vi "While Loop Stop with Nested Conditionals Example.vi"() -> ()   [LabVIEW 2020, in "Test Executive.lvlib" / "Nested Conditional in While Loop Example.lvlib"]
uses:
  <vilib>/gpm_packages/@cs/test-executive/Source/Sandbox/Nested Conditional in While Loop Example/Nested Conditional in While Loop Example.lvlib
  <vilib>/gpm_packages/@cs/test-executive/Source/Test Executive/TestExecutive/Test Executive.lvclass
  C:/Program Files/National Instruments/LabVIEW 2020/vi.lib/gpm_packages/@cs/test-executive/Source/Test Executive/ITestExecutive/ITest Executive.lvclass
  <vilib>/gpm_packages/@cs/test-executive/Source/Sandbox/Nested Conditional in While Loop Example/Device End Finder/Device End Finder.lvclass
  <vilib>/gpm_packages/@cs/test-executive/Source/Sandbox/Nested Conditional in While Loop Example/iTest Step/iTest Step.lvclass
  <vilib>/gpm_packages/@cs/test-executive/Source/Sandbox/Nested Conditional in While Loop Example/Device Post Dip Length/Device Post Dip Length.lvclass
  <vilib>/gpm_packages/@cs/test-executive/Source/Sandbox/Nested Conditional in While Loop Example/Iterate/Iterate.lvclass
  <vilib>/gpm_packages/@cs/run-time-assertions/Source/Assert Less/Assert Less.lvclass
  C:/Program Files/National Instruments/LabVIEW 2020/vi.lib/gpm_packages/@cs/run-time-assertions/Source/Assert/Assert.lvclass
  <vilib>/gpm_packages/@cs/run-time-assertions/Source/Assert Greater or Equal/Assert Greater or Equal.lvclass
  52cc7c55-fdef-40cb-9b01-06c8b27f6ce0.vi
  a0d94dfd-d8d0-4b1a-8204-38a80b6efbaa.vi
  22f6ace6-23ce-4251-a6e4-277f1b0ddc71.vi
  5f10894d-39a4-4711-8d45-a7dfc19e406e.vi
  be74f702-6a90-4609-b438-3fe557b35d77.vi
  a10d8200-898b-41a6-a462-7d6528bd6408.vi
  f7a3b14d-821f-4fd9-982f-4d6d978a7b0b.vi
  0ece8d78-e94c-4796-b66e-215c9e74c0e8.vi
  0df7ce8f-9091-4b2d-8a2a-2bb6b5b20627.vi
  b94ec968-1831-4c86-b0ad-5031bb25da7e.vi
  78029b1d-24e3-44ce-bc53-a6c931d15c9f.vi
  <vilib>/Utility/error.llb/Error Cluster From Error Code.vi
  <vilib>/gpm_packages/@cs/test-executive/Source/Test Executive/ITestExecutive/ITest Executive.lvclass
  <vilib>/gpm_packages/@cs/test-executive/Source/Test Executive/TestExecutive Ref/TestExecutive Ref.lvclass
  <vilib>/gpm_packages/@cs/test-executive/Source/Test Executive/Executioner/Executioner.lvclass
panel:
  in  "Stop":bool
  in  "Tree":string(tree)
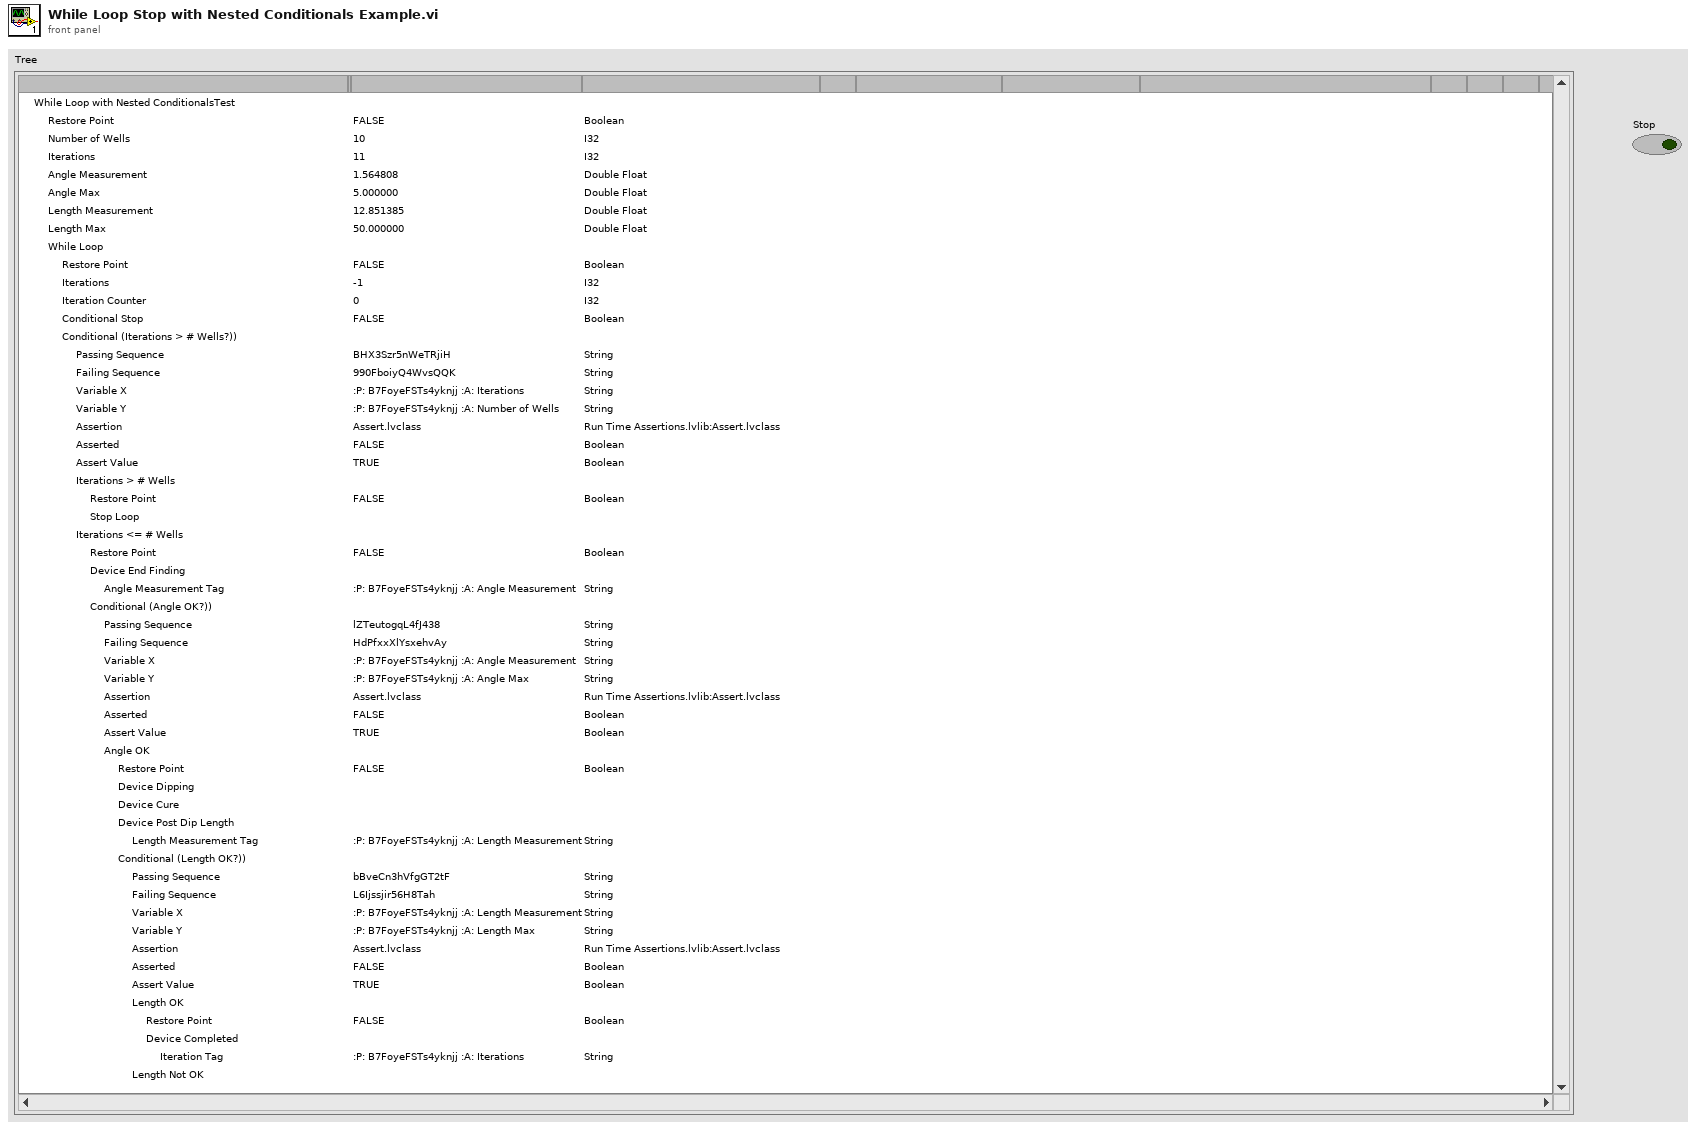
[diagram p1: front panel]
types:
  T1 = cluster{"Left Cell String":string, "Child Text":string[], "Child Tag":string, "Item Indent":i32, "Child Only?":bool, "Glyph Index":i32}[]
diagram:
  n1 = flat-sequence {
    tunnel: [w184] -> w181
    tunnel: [w183] -> w180
    tunnel: [w182] -> w168
    frame #0 {
      # "Create Test Executive"
      n2 = call <vilib>:"Create New Test Executive.vi"("Name"="While Loop with Nested ConditionalsTest", "Test Executive"=refnum<class "Test Executive.lvclass"> refnum ("Test Executive.lvlib:Test Executive.lvclass")) -> ("error out"=w183:errorcluster, "Test Executive Ref"=w184:refnum<data-value>, "Test Executive ID out"=w182:string)  [unwired: 7 in]
    }
  }
  n3 = flat-sequence {
    tunnel: w181 -> [w198]
    tunnel: w180 -> [w197]
    tunnel: [w191] -> w165
    tunnel: [w190] -> w166
    tunnel: [w189] -> w170
    tunnel: [w188] -> w169
    tunnel: w168 -> [w187]
    tunnel: [w187] -> w167
    frame #0 {
      # "Create attributes for stopping top level loop"
      n4 = call "Add Attribute.vim"("ID"=w187, "error in (no error)"=w197, "Attribute"=10, "Attribute Name"="Number of Wells", "Test Executive Ref"=w198) -> ("error out"=w192:errorcluster, "Attribute ID out"=w191:string, "Test Executive Ref out"=w193:refnum<data-value>)  [unwired: 3 in, 1 out]
      n5 = call "Add Attribute.vim"("ID"=w187, "error in (no error)"=w192, "Attribute"=0, "Attribute Name"="Iterations", "Test Executive Ref"=w193) -> ("error out"=w188:errorcluster, "Attribute ID out"=w190:string, "Test Executive Ref out"=w189:refnum<data-value>)  [unwired: 3 in, 1 out]
    }
  }
  n6 = flat-sequence {
    tunnel: w170 -> [w212]
    tunnel: [w205] -> w159
    tunnel: w169 -> [w211]
    tunnel: [w203] -> w157
    tunnel: w167 -> [w202]
    tunnel: [w202] -> w164
    tunnel: [w210] -> w162
    tunnel: w166 -> [w210]
    tunnel: [w209] -> w163
    tunnel: w165 -> [w209]
    tunnel: [w201] -> w161
    tunnel: [w200] -> w160
    frame #0 {
      # "Create attributes for Angle OK evaluation\nNote that we are just creating a made up Angle Max that we can use for comparison purposes in the conditional"
      n7 = call "Add Attribute.vim"("ID"=w202, "error in (no error)"=w211, "Attribute"=0.0, "Attribute Name"="Angle Measurement", "Test Executive Ref"=w212) -> ("error out"=w204:errorcluster, "Attribute ID out"=w201:string, "Test Executive Ref out"=w206:refnum<data-value>)  [unwired: 3 in, 1 out]
      n8 = call "Add Attribute.vim"("ID"=w202, "error in (no error)"=w204, "Attribute"=5.0, "Attribute Name"="Angle Max", "Test Executive Ref"=w206) -> ("error out"=w203:errorcluster, "Attribute ID out"=w200:string, "Test Executive Ref out"=w205:refnum<data-value>)  [unwired: 3 in, 1 out]
    }
  }
  n9 = flat-sequence {
    tunnel: [w226] -> w158
    tunnel: [w224] -> w156
    tunnel: [w221] -> w155
    tunnel: [w219] -> w154
    tunnel: [w220] -> w153
    tunnel: [w223] -> w150
    tunnel: [w222] -> w149
    tunnel: w164 -> [w221]
    tunnel: w163 -> [w220]
    tunnel: w162 -> [w219]
    tunnel: [w218] -> w152
    tunnel: w161 -> [w218]
    tunnel: [w217] -> w151
    tunnel: w160 -> [w217]
    tunnel: w159 -> [w216]
    tunnel: w157 -> [w215]
    frame #0 {
      # "Create attributes for Length OK evaluation\nNote that we are just creating a made up Length Max that we can use for comparison purposes in the conditional"
      n10 = call "Add Attribute.vim"("ID"=w221, "error in (no error)"=w215, "Attribute"=0.0, "Attribute Name"="Length Measurement", "Test Executive Ref"=w216) -> ("error out"=w225:errorcluster, "Attribute ID out"=w223:string, "Test Executive Ref out"=w227:refnum<data-value>)  [unwired: 3 in, 1 out]
      n11 = call "Add Attribute.vim"("ID"=w221, "error in (no error)"=w225, "Attribute"=50.0, "Attribute Name"="Length Max", "Test Executive Ref"=w227) -> ("error out"=w224:errorcluster, "Attribute ID out"=w222:string, "Test Executive Ref out"=w226:refnum<data-value>)  [unwired: 3 in, 1 out]
    }
  }
  n12 = flat-sequence {
    tunnel: [w243] -> w179
    tunnel: [w242] -> w178
    tunnel: [w241] -> w145
    tunnel: w155 -> [w232]
    tunnel: w158 -> [w240]
    tunnel: w156 -> [w239]
    tunnel: [w232] -> w148
    tunnel: [w238] -> w147
    tunnel: w154 -> [w238]
    tunnel: [w237] -> w146
    tunnel: w153 -> [w237]
    tunnel: w152 -> [w236]
    tunnel: w151 -> [w235]
    tunnel: w150 -> [w234]
    tunnel: w149 -> [w233]
    tunnel: [w236] -> w141
    tunnel: [w235] -> w142
    tunnel: [w234] -> w143
    tunnel: [w233] -> w144
    frame #0 {
      # "Create While Loop"
      n13 = call <vilib>:"Insert While Loop.vi"("Parent ID"=w232, "error in (no error)"=w239, "Name"="While Loop", "Test Executive Ref"=w240) -> ("error out"=w242:errorcluster, "Test Executive Ref out"=w243:refnum<data-value>, "Unique ID out"=w241:string)  [unwired: 4 in, 1 out]
    }
  }
  n14 = flat-sequence {
    tunnel: w179 -> [w261]
    tunnel: w178 -> [w260]
    tunnel: w145 -> [w249]
    tunnel: [w257] -> w177
    tunnel: [w255] -> w176
    tunnel: [w254] -> w138
    tunnel: [w252] -> w140
    tunnel: w148 -> [w252]
    tunnel: [w251] -> w136
    tunnel: w147 -> [w251]
    tunnel: w146 -> [w250]
    tunnel: [w250] -> w137
    tunnel: [w249] -> w139
    tunnel: [w248] -> w132
    tunnel: w144 -> [w248]
    tunnel: [w247] -> w133
    tunnel: w143 -> [w247]
    tunnel: [w246] -> w134
    tunnel: w142 -> [w246]
    tunnel: [w245] -> w135
    tunnel: w141 -> [w245]
    frame #0 {
      # "Create True Conditional Branch and nest a Stop Loop\nThis branch executes when Iterations > # wells"
      n15 = call <vilib>:"Insert Conditional Branch.vi"("Parent ID"=w249, "error in (no error)"=w260, "Name"="Iterations > # Wells", "Test Executive Ref"=w261) -> ("error out"=w256:errorcluster, "Test Executive Ref out"=w258:refnum<data-value>, "Unique ID out"=w254:string)  [unwired: 4 in, 1 out]
      n16 = call <vilib>:"Insert Stop Loop.vi"("Parent ID"=w254, "error in (no error)"=w256, "Name"="Stop Loop", "Test Executive Ref"=w258) -> ("error out"=w255:errorcluster, "Test Executive Ref out"=w257:refnum<data-value>)  [unwired: 4 in, 2 out]
    }
  }
  n17 = flat-sequence {
    tunnel: w177 -> [w275]
    tunnel: w176 -> [w274]
    tunnel: [w263] -> w70
    tunnel: [w262] -> w69
    tunnel: [w273] -> w71
    tunnel: w139 -> [w271]
    tunnel: [w272] -> w73
    tunnel: w140 -> [w272]
    tunnel: [w271] -> w72
    tunnel: [w270] -> w62
    tunnel: w138 -> [w270]
    tunnel: w137 -> [w269]
    tunnel: [w269] -> w63
    tunnel: [w268] -> w64
    tunnel: w136 -> [w268]
    tunnel: [w267] -> w65
    tunnel: w135 -> [w267]
    tunnel: [w266] -> w66
    tunnel: w134 -> [w266]
    tunnel: [w265] -> w67
    tunnel: w133 -> [w265]
    tunnel: [w264] -> w68
    tunnel: w132 -> [w264]
    frame #0 {
      # "Create False Conditional Branch\nThis branch exectues when Iterations <= # Wells"
      n18 = call <vilib>:"Insert Conditional Branch.vi"("Parent ID"=w271, "error in (no error)"=w274, "Name"="Iterations <= # Wells", "Test Executive Ref"=w275) -> ("error out"=w262:errorcluster, "Test Executive Ref out"=w263:refnum<data-value>, "Unique ID out"=w273:string)  [unwired: 4 in, 1 out]
    }
  }
  n19 = flat-sequence {
    tunnel: w70 -> [w294]
    tunnel: [w293] -> w129
    tunnel: w69 -> [w292]
    tunnel: [w291] -> w128
    tunnel: w71 -> [w287]
    tunnel: [w289] -> w123
    tunnel: w73 -> [w289]
    tunnel: [w288] -> w122
    tunnel: w72 -> [w288]
    tunnel: [w287] -> w130
    tunnel: [w286] -> w120
    tunnel: w64 -> [w286]
    tunnel: [w285] -> w119
    tunnel: w63 -> [w285]
    tunnel: [w284] -> w118
    tunnel: w62 -> [w284]
    tunnel: w65 -> [w283]
    tunnel: w66 -> [w282]
    tunnel: w67 -> [w281]
    tunnel: w68 -> [w280]
    tunnel: [w283] -> w124
    tunnel: [w282] -> w125
    tunnel: [w281] -> w126
    tunnel: [w280] -> w127
    tunnel: [w277] -> w131
    frame #0 {
      # "Device End Finding\nThis should generate an Angle measurement"
      n20 = call <vilib>:"Create Test from Object.vi"("Test"=refnum<class "Device End Finder.lvclass"> refnum ("Nested Conditional in While Loop Example.lvlib:Device End Finder.lvclass")) -> ("Test"=w279:refnum<class "Executioner.lvclass">)  [unwired: 10 in]
      n21 = call <vilib>:"Insert Test.vi"("Parent ID"=w287, "error in (no error)"=w292, "Test"=w279, "Name"="Device End Finding", "Test Executive Ref"=w294) -> ("error out"=w291:errorcluster, "Test Executive Ref out"=w293:refnum<data-value>, "Unique ID out"=w277:string)  [unwired: 3 in, 1 out]
    }
  }
  n22 = flat-sequence {
    tunnel: w129 -> [w310]
    tunnel: w128 -> [w309]
    tunnel: w131 -> [w308]
    tunnel: [w306] -> _
    tunnel: [w305] -> _
    tunnel: w120 -> [w299]
    tunnel: [w304] -> _
    tunnel: w123 -> [w304]
    tunnel: [w296] -> _
    tunnel: [w296] -> _
    tunnel: [w303] -> w121
    tunnel: w130 -> [w303]
    tunnel: [w302] -> w114
    tunnel: w127 -> [w302]
    tunnel: [w301] -> w115
    tunnel: w126 -> [w301]
    tunnel: [w300] -> w116
    tunnel: w125 -> [w300]
    tunnel: w124 -> [w295]
    tunnel: [w299] -> _
    tunnel: [w298] -> _
    tunnel: w118 -> [w298]
    tunnel: [w297] -> _
    tunnel: w119 -> [w297]
    tunnel: [w295] -> w117
    tunnel: w122 -> [w296]
    frame #0 {
      # "Insert an attribute that holds the\ntag for the variable we want to\nstore angle measurement in"
      n23 = call "Add Attribute.vim"("ID"=w308, "error in (no error)"=w309, "Attribute"=w295, "Attribute Name"="Angle Measurement Tag", "Test Executive Ref"=w310) -> ("error out"=w305:errorcluster, "Test Executive Ref out"=w306:refnum<data-value>)  [unwired: 3 in, 2 out]
    }
  }
  n24 = flat-sequence {
    tunnel: [w318] -> w109
    tunnel: [w315] -> w108
    tunnel: w121 -> [w331]
    tunnel: w129 -> [w335]
    tunnel: w128 -> [w334]
    tunnel: [w333] -> w113
    tunnel: w123 -> [w333]
    tunnel: [w332] -> w112
    tunnel: w122 -> [w332]
    tunnel: [w331] -> w111
    tunnel: [w330] -> w105
    tunnel: w120 -> [w330]
    tunnel: w119 -> [w311]
    tunnel: [w329] -> w107
    tunnel: w118 -> [w329]
    tunnel: [w328] -> w104
    tunnel: w117 -> [w328]
    tunnel: [w327] -> w103
    tunnel: w116 -> [w327]
    tunnel: [w326] -> w102
    tunnel: w115 -> [w326]
    tunnel: [w325] -> w101
    tunnel: w114 -> [w325]
    tunnel: [w314] -> w110
    tunnel: [w311] -> w106
    frame #0 {
      # "This branch executes when Angle measurement after Device End Finding returns as OK\nInsert some dummy test steps that match the flow chart"
      n25 = call <vilib>:"Insert Conditional Branch.vi"("Parent ID"=w331, "error in (no error)"=w334, "Name"="Angle OK", "Test Executive Ref"=w335) -> ("error out"=w317:errorcluster, "Test Executive Ref out"=w320:refnum<data-value>, "Unique ID out"=w314:string)  [unwired: 4 in, 1 out]
      n26 = call <vilib>:"Create Test from Object.vi"("Test"=refnum<class "iTest Step.lvclass"> refnum ("Nested Conditional in While Loop Example.lvlib:iTest Step.lvclass")) -> ("Test"=w324:refnum<class "Executioner.lvclass">)  [unwired: 10 in]
      n27 = call <vilib>:"Insert Test.vi"("Parent ID"=w314, "error in (no error)"=w317, "Test"=w324, "Name"="Device Dipping", "Test Executive Ref"=w320) -> ("error out"=w316:errorcluster, "Test Executive Ref out"=w319:refnum<data-value>)  [unwired: 3 in, 2 out]
      n28 = call <vilib>:"Create Test from Object.vi"("Test"=refnum<class "iTest Step.lvclass"> refnum ("Nested Conditional in While Loop Example.lvlib:iTest Step.lvclass")) -> ("Test"=w321:refnum<class "Executioner.lvclass">)  [unwired: 10 in]
      n29 = call <vilib>:"Insert Test.vi"("Parent ID"=w314, "error in (no error)"=w316, "Test"=w321, "Name"="Device Cure", "Test Executive Ref"=w319) -> ("error out"=w315:errorcluster, "Test Executive Ref out"=w318:refnum<data-value>)  [unwired: 3 in, 2 out]
    }
  }
  n30 = flat-sequence {
    tunnel: w109 -> [w355]
    tunnel: [w354] -> w95
    tunnel: w108 -> [w353]
    tunnel: [w352] -> w94
    tunnel: w111 -> [w340]
    tunnel: [w350] -> w100
    tunnel: w113 -> [w350]
    tunnel: [w349] -> w99
    tunnel: w112 -> [w349]
    tunnel: [w340] -> w98
    tunnel: [w348] -> w89
    tunnel: w105 -> [w348]
    tunnel: [w347] -> w88
    tunnel: w106 -> [w347]
    tunnel: [w346] -> w87
    tunnel: w107 -> [w346]
    tunnel: w104 -> [w345]
    tunnel: w103 -> [w344]
    tunnel: w102 -> [w343]
    tunnel: w101 -> [w342]
    tunnel: [w345] -> w90
    tunnel: [w344] -> w91
    tunnel: [w343] -> w92
    tunnel: [w342] -> w93
    tunnel: w110 -> [w339]
    tunnel: [w339] -> w97
    tunnel: [w338] -> w96
    frame #0 {
      # "Device End Finding\nThis should generate an Angle measurement"
      n31 = call <vilib>:"Create Test from Object.vi"("Test"=refnum<class "Device Post Dip Length.lvclass"> refnum ("Nested Conditional in While Loop Example.lvlib:Device Post Dip Length.lvclass")) -> ("Test"=w341:refnum<class "Executioner.lvclass">)  [unwired: 10 in]
      n32 = call <vilib>:"Insert Test.vi"("Parent ID"=w339, "error in (no error)"=w353, "Test"=w341, "Name"="Device Post Dip Length", "Test Executive Ref"=w355) -> ("error out"=w352:errorcluster, "Test Executive Ref out"=w354:refnum<data-value>, "Unique ID out"=w338:string)  [unwired: 3 in, 1 out]
    }
  }
  n33 = flat-sequence {
    tunnel: [w372] -> w86
    tunnel: w100 -> [w372]
    tunnel: [w371] -> w85
    tunnel: w99 -> [w371]
    tunnel: [w370] -> w84
    tunnel: w98 -> [w370]
    tunnel: [w358] -> w83
    tunnel: w97 -> [w358]
    tunnel: [w362] -> w82
    tunnel: w95 -> [w363]
    tunnel: [w360] -> w81
    tunnel: w94 -> [w361]
    tunnel: [w369] -> w74
    tunnel: w93 -> [w369]
    tunnel: [w357] -> w75
    tunnel: w92 -> [w357]
    tunnel: w91 -> [w368]
    tunnel: [w368] -> w76
    tunnel: w90 -> [w367]
    tunnel: [w367] -> w77
    tunnel: [w366] -> w80
    tunnel: w87 -> [w366]
    tunnel: [w365] -> w79
    tunnel: w88 -> [w365]
    tunnel: [w364] -> w78
    tunnel: w89 -> [w364]
    tunnel: w96 -> [w356]
    frame #0 {
      # "Insert an attribute that holds the\ntag for the variable we want to\nstore length measurement in"
      n34 = call "Add Attribute.vim"("ID"=w356, "error in (no error)"=w361, "Attribute"=w357, "Attribute Name"="Length Measurement Tag", "Test Executive Ref"=w363) -> ("error out"=w360:errorcluster, "Test Executive Ref out"=w362:refnum<data-value>)  [unwired: 3 in, 2 out]
    }
  }
  n35 = flat-sequence {
    tunnel: [w398] -> w51
    tunnel: w86 -> [w398]
    tunnel: [w397] -> w50
    tunnel: w85 -> [w397]
    tunnel: [w387] -> w49
    tunnel: w84 -> [w387]
    tunnel: w83 -> [w376]
    tunnel: w82 -> [w393]
    tunnel: w81 -> [w392]
    tunnel: [w378] -> w54
    tunnel: w78 -> [w378]
    tunnel: [w396] -> w53
    tunnel: w79 -> [w396]
    tunnel: [w395] -> w52
    tunnel: w80 -> [w395]
    tunnel: w77 -> [w384]
    tunnel: w76 -> [w385]
    tunnel: w75 -> [w377]
    tunnel: w74 -> [w386]
    tunnel: [w386] -> w58
    tunnel: [w377] -> w57
    tunnel: [w385] -> w56
    tunnel: [w384] -> w55
    tunnel: [w376] -> w61
    tunnel: [w375] -> w60
    tunnel: [w374] -> w59
    tunnel: [w373] -> w43
    frame #0 {
      # "This is the branch that will execute when the length measurement is OK.\nIt will call the Device Completed test step, which runs a dummy step that will increment the counter"
      n36 = call <vilib>:"Insert Conditional Branch.vi"("Parent ID"=w376, "error in (no error)"=w392, "Name"="Length OK", "Test Executive Ref"=w393) -> ("error out"=w388:errorcluster, "Test Executive Ref out"=w389:refnum<data-value>, "Unique ID out"=w373:string)  [unwired: 4 in, 1 out]
      n37 = call <vilib>:"Create Test from Object.vi"("Test"=refnum<class "Iterate.lvclass"> refnum ("Nested Conditional in While Loop Example.lvlib:Iterate.lvclass")) -> ("Test"=w390:refnum<class "Executioner.lvclass">)  [unwired: 10 in]
      n38 = call <vilib>:"Insert Test.vi"("Parent ID"=w373, "error in (no error)"=w388, "Test"=w390, "Name"="Device Completed", "Test Executive Ref"=w389) -> ("error out"=w380:errorcluster, "Test Executive Ref out"=w381:refnum<data-value>, "Unique ID out"=w379:string)  [unwired: 3 in, 1 out]
      n39 = call "Add Attribute.vim"("ID"=w379, "error in (no error)"=w380, "Attribute"=w378, "Attribute Name"="Iteration Tag", "Test Executive Ref"=w381) -> ("error out"=w374:errorcluster, "Test Executive Ref out"=w375:refnum<data-value>)  [unwired: 3 in, 2 out]
    }
  }
  n40 = flat-sequence {
    tunnel: [w425] -> w40
    tunnel: w51 -> [w425]
    tunnel: [w424] -> w39
    tunnel: w50 -> [w424]
    tunnel: [w414] -> w38
    tunnel: w49 -> [w414]
    tunnel: w61 -> [w403]
    tunnel: w60 -> [w420]
    tunnel: w59 -> [w419]
    tunnel: [w405] -> w35
    tunnel: w54 -> [w405]
    tunnel: [w423] -> w34
    tunnel: w53 -> [w423]
    tunnel: [w422] -> w33
    tunnel: w52 -> [w422]
    tunnel: w55 -> [w411]
    tunnel: w56 -> [w412]
    tunnel: w57 -> [w404]
    tunnel: w58 -> [w413]
    tunnel: [w413] -> w47
    tunnel: [w404] -> w48
    tunnel: [w412] -> w37
    tunnel: [w411] -> w36
    tunnel: [w403] -> w44
    tunnel: [w402] -> w46
    tunnel: [w401] -> w45
    tunnel: w43 -> [w400]
    tunnel: [w400] -> w42
    tunnel: [w399] -> w41
    frame #0 {
      # "This is the branch that will execute when the length measurement is not OK.\nIt will call the Device Rejection test step, which runs a dummy step that will increment the counter"
      n41 = call <vilib>:"Insert Conditional Branch.vi"("Parent ID"=w403, "error in (no error)"=w419, "Name"="Length Not OK", "Test Executive Ref"=w420) -> ("error out"=w415:errorcluster, "Test Executive Ref out"=w416:refnum<data-value>, "Unique ID out"=w399:string)  [unwired: 4 in, 1 out]
      n42 = call <vilib>:"Create Test from Object.vi"("Test"=refnum<class "Iterate.lvclass"> refnum ("Nested Conditional in While Loop Example.lvlib:Iterate.lvclass")) -> ("Test"=w417:refnum<class "Executioner.lvclass">)  [unwired: 10 in]
      n43 = call <vilib>:"Insert Test.vi"("Parent ID"=w399, "error in (no error)"=w415, "Test"=w417, "Name"="Device Rejection", "Test Executive Ref"=w416) -> ("error out"=w407:errorcluster, "Test Executive Ref out"=w408:refnum<data-value>, "Unique ID out"=w406:string)  [unwired: 3 in, 1 out]
      n44 = call "Add Attribute.vim"("ID"=w406, "error in (no error)"=w407, "Attribute"=w405, "Attribute Name"="Iteration Tag", "Test Executive Ref"=w408) -> ("error out"=w401:errorcluster, "Test Executive Ref out"=w402:refnum<data-value>)  [unwired: 3 in, 2 out]
    }
  }
  n45 = flat-sequence {
    tunnel: w48 -> [w443]
    tunnel: w47 -> [w442]
    tunnel: w46 -> [w440]
    tunnel: w45 -> [w439]
    tunnel: w44 -> [w426]
    tunnel: w42 -> [w438]
    tunnel: w41 -> [w437]
    tunnel: [w436] -> w32
    tunnel: w40 -> [w436]
    tunnel: [w435] -> w31
    tunnel: w39 -> [w435]
    tunnel: [w434] -> w30
    tunnel: w38 -> [w434]
    tunnel: w37 -> [w433]
    tunnel: w36 -> [w432]
    tunnel: [w433] -> w27
    tunnel: [w432] -> w26
    tunnel: [w431] -> w23
    tunnel: w35 -> [w431]
    tunnel: w34 -> [w430]
    tunnel: [w430] -> w24
    tunnel: w33 -> [w429]
    tunnel: [w429] -> w25
    tunnel: [w428] -> w29
    tunnel: [w427] -> w28
    tunnel: [w426] -> w22
    frame #0 {
      # "Setup the conditional inside the Length OK Branch"
      n46 = call <vilib>:"Insert Conditional.vi"("Test Executive Ref"=w440, "Name"="Conditional (Length OK?))", "Assertion"=refnum<class "Assert Less.lvclass"> refnum ("Run Time Assertions.lvlib:Assert Less.lvclass"), "error in (no error)"=w439, "Parent ID"=w426, "Variable X"=w443, "Variable Y"=w442, "Passing Executive"=w438, "Failing Executive"=w437) -> ("Test Executive Ref out"=w428:refnum<data-value>, "error out"=w427:errorcluster)  [unwired: 7 in, 2 out]
    }
  }
  n47 = flat-sequence {
    tunnel: [w449] -> w20
    tunnel: [w447] -> w18
    tunnel: w30 -> [w461]
    tunnel: [w463] -> w13
    tunnel: w32 -> [w463]
    tunnel: [w462] -> w12
    tunnel: w31 -> [w462]
    tunnel: [w461] -> w10
    tunnel: w29 -> [w460]
    tunnel: w28 -> [w459]
    tunnel: w27 -> [w453]
    tunnel: w26 -> [w454]
    tunnel: [w458] -> w9
    tunnel: w25 -> [w458]
    tunnel: [w457] -> w8
    tunnel: w24 -> [w457]
    tunnel: w23 -> [w445]
    tunnel: [w445] -> w6
    tunnel: w22 -> [w456]
    tunnel: [w456] -> w15
    tunnel: [w455] -> w14
    tunnel: [w454] -> w17
    tunnel: [w453] -> w16
    frame #0 {
      # "This branch executes when Angle measurement after Device End Finding returns as Not OK"
      n48 = call <vilib>:"Insert Conditional Branch.vi"("Parent ID"=w461, "error in (no error)"=w459, "Name"="Angle Not OK", "Test Executive Ref"=w460) -> ("error out"=w466:errorcluster, "Test Executive Ref out"=w467:refnum<data-value>, "Unique ID out"=w455:string)  [unwired: 4 in, 1 out]
      n49 = call <vilib>:"Create Test from Object.vi"("Test"=refnum<class "Iterate.lvclass"> refnum ("Nested Conditional in While Loop Example.lvlib:Iterate.lvclass")) -> ("Test"=w464:refnum<class "Executioner.lvclass">)  [unwired: 10 in]
      n50 = call <vilib>:"Insert Test.vi"("Parent ID"=w455, "error in (no error)"=w466, "Test"=w464, "Name"="Device Rejection", "Test Executive Ref"=w467) -> ("error out"=w448:errorcluster, "Test Executive Ref out"=w450:refnum<data-value>, "Unique ID out"=w446:string)  [unwired: 3 in, 1 out]
      n51 = call "Add Attribute.vim"("ID"=w446, "error in (no error)"=w448, "Attribute"=w445, "Attribute Name"="Iteration Tag", "Test Executive Ref"=w450) -> ("error out"=w447:errorcluster, "Test Executive Ref out"=w449:refnum<data-value>)  [unwired: 3 in, 2 out]
    }
  }
  n52 = flat-sequence {
    tunnel: [w482] -> w21
    tunnel: w20 -> [w481]
    tunnel: [w480] -> w19
    tunnel: w18 -> [w479]
    tunnel: w10 -> [w472]
    tunnel: w17 -> [w478]
    tunnel: w16 -> [w477]
    tunnel: w15 -> [w476]
    tunnel: w14 -> [w475]
    tunnel: [w474] -> w2
    tunnel: w13 -> [w474]
    tunnel: w12 -> [w473]
    tunnel: [w473] -> w11
    tunnel: [w472] -> w3
    tunnel: [w471] -> w4
    tunnel: w9 -> [w471]
    tunnel: [w470] -> w7
    tunnel: w8 -> [w470]
    tunnel: w6 -> [w469]
    tunnel: [w469] -> w5
    frame #0 {
      # "Setup the conditional inside the Angle OK Branch"
      n53 = call <vilib>:"Insert Conditional.vi"("Test Executive Ref"=w481, "Name"="Conditional (Angle OK?))", "Assertion"=refnum<class "Assert Less.lvclass"> refnum ("Run Time Assertions.lvlib:Assert Less.lvclass"), "error in (no error)"=w479, "Parent ID"=w472, "Variable X"=w478, "Variable Y"=w477, "Passing Executive"=w476, "Failing Executive"=w475) -> ("Test Executive Ref out"=w482:refnum<data-value>, "error out"=w480:errorcluster)  [unwired: 7 in, 2 out]
    }
  }
  n54 = flat-sequence {
    tunnel: [w495] -> w175
    tunnel: [w494] -> w174
    tunnel: w21 -> [w493]
    tunnel: w19 -> [w492]
    tunnel: w11 -> [w491]
    tunnel: w7 -> [w490]
    tunnel: w5 -> [w489]
    tunnel: w4 -> [w486]
    tunnel: w3 -> [w487]
    tunnel: [w488] -> w1
    tunnel: w2 -> [w488]
    frame #0 {
      # "Create the Conditional Structure\nthat decides if Iterations > Number of wells and stops the While Loop"
      n55 = call <vilib>:"Insert Conditional.vi"("Test Executive Ref"=w493, "Name"="Conditional (Iterations > # Wells?))", "Assertion"=refnum<class "Assert Greater or Equal.lvclass"> refnum ("Run Time Assertions.lvlib:Assert Greater or Equal.lvclass"), "error in (no error)"=w492, "Parent ID"=w491, "Variable X"=w489, "Variable Y"=w490, "Passing Executive"=w486, "Failing Executive"=w487) -> ("Test Executive Ref out"=w495:refnum<data-value>, "error out"=w494:errorcluster)  [unwired: 7 in, 2 out]
    }
  }
  n56 = control-ref of="Tree"() -> (w173:refnum<vi>)
  n57 = while {
    shift-right: [w516] -> w172
    shift-left: w175 -> [w514]
    shift-right: [w515] -> w171
    shift-left: w174 -> [w512]
    tunnel: w1 -> [w510]
    shift-right: [w500] -> _
    shift-left: w1 -> [w503]
    tunnel: w173 -> [w509]
    stop <- w499 stop-if-true
    # "Draw the Tree & Run the Get Next"
    n58 = invoke on="Invoke Node" class="Tree (strict)" method="Edit Tree Items.Delete"(reference=w509) -> (reference out=w508:refnum<vi>)  [unwired: 4 in, 4 out]
    n59 = call <vilib>:"Build Tree Data Type.vi"("Show IDs (True)"=FALSE, "Test ID"=w510, "error in (no error)"=w512, "Test Executive Ref"=w514) -> ("error out"=w511:errorcluster, "Tree Data"=w507:T1, "Test Executive Ref out"=w513:refnum<data-value>)  [unwired: 5 in]
    n60 = invoke on="Invoke Node" class="Tree (strict)" method="Edit Tree Items.Add Multiple Items to End"(reference=w508, "Items"=w507) -> (reference out=w504:refnum<vi>)  [unwired: 2 in, 3 out]
    n61 = property on="Property Node" class="Tree (strict)"(reference=w504, "Active Item Tag"=w503, "CellBG"=u32 16777226) -> (reference out=w501:refnum<vi>)  [unwired: 1 in, 1 out]
    n62 = call <vilib>:"Get Next.vi"("error in (no error)"=w511, "Test Executive Ref"=w513) -> ("error out"=w517:errorcluster, "Test"=w518:refnum<class "Executioner.lvclass">, "Test Executive Ref out"=w519:refnum<data-value>, "Found"=w520:bool, "Unique ID out"=w500:string, "Complete"=w521:bool)  [unwired: 3 in, 1 out]
    n63 = Or(x=w521, y="Stop") -> (x .or. y?=w499:bool)
    n64 = property on="Property Node" class="Tree (strict)"(reference=w501, "Active Item Tag"=w500, "CellBG"=u32 14125311) -> ()  [unwired: 1 in, 2 out]
    n65 = case shown="False" w521 {
      tunnel: w520 -> [w527 _]
      tunnel: w519 -> [w526 w535]
      tunnel: w518 -> [w525 _]
      tunnel: w517 -> [w524 w534]
      tunnel: [w523 w535] -> w516
      tunnel: [w522 w534] -> w515
      frame False {
        # "Executioner is not complete"
        n66 = case shown="True" w527 {
          tunnel: w526 -> [w529 w532]
          tunnel: w525 -> [_ w533]
          tunnel: w524 -> [w528 w531]
          tunnel: [w529 w532] -> w523
          tunnel: [w528 w530] -> w522
          frame False {
            # "This is not an executioner, don't do that thang..."
          }
          frame True {
            # "This is an executioner.  Do That Thang..."
            n67 = call <vilib>:"Do That Thang.vi"("Test Executive Ref out"=w532, "error in (no error)"=w531, "Executioner in"=w533) -> ("error out"=w530:errorcluster)  [unwired: 8 in]
          }
        }
      }
      frame True {
        # "Executioner is complete, stop"
      }
    }
    n68 = Wait (ms)(milliseconds to wait=u32 1000) -> ()  [unwired: 1 out]
  }
  n69 = call <vilib>:"Destroy Test Executive.vi"("error in (no error)"=w171, "Test Executive Ref"=w172) -> ()  [unwired: 9 in, 1 out]
